vi "Open serial.vi"(8 "error in (no error)":errorcluster, 10 "port":string, 11 "Roda_Filtros in":refnum<class "Roda_Filtros.lvclass">) -> (0 "error out":errorcluster, 2 "status":bool, 3 "Roda_Filtros out":refnum<class "Roda_Filtros.lvclass">)   [LabVIEW 2018, in "Roda_Filtros.lvclass"]
uses:
  Roda_Filtros.lvclass
  Roda_Filtros.lvclass/Roda_Filtros.ctl
  <vilib>/Instr/_visa.llb/VISA Configure Serial Port (Instr).vi
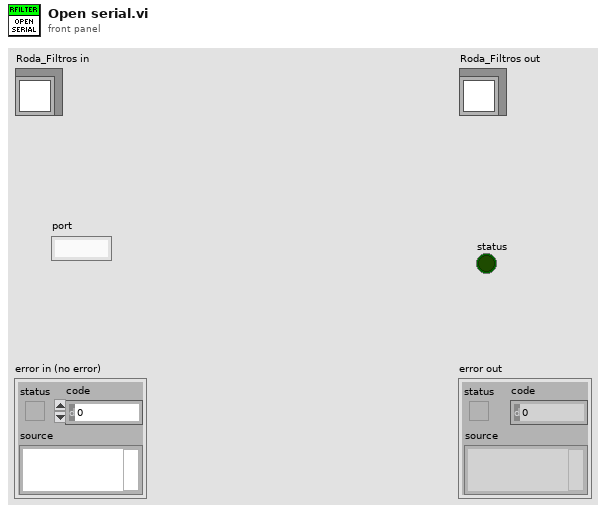
[diagram p1: front panel]
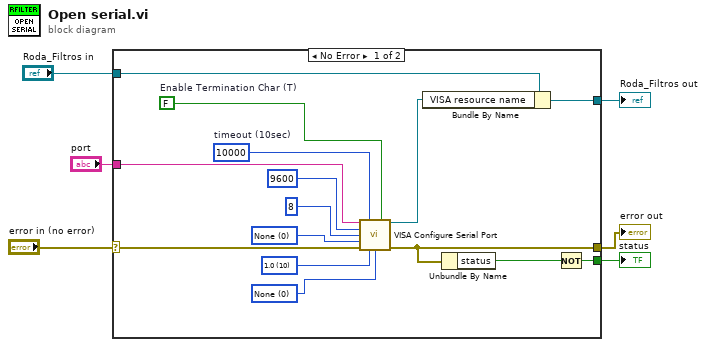
[diagram p0: block diagram]
diagram:
  n1 = case shown="No Error" "error in (no error)" {
    selector: "error in (no error)" -> [w14 w23]
    tunnel: [w9 w23] -> w5
    tunnel: [w12 w22] -> w3
    tunnel: "Roda_Filtros in" -> [w13 w22]
    tunnel: "port" -> [w10 _]
    tunnel: [w7 _] -> w1
    frame No Error {
      w20 = u16 0 items=["None", "Odd", "Even", "Mark", "Space"] ("parity")
      w17 = u16 10 items=["1.0"=10, "1.5"=15, "2.0"=20] ("stop bits")
      w16 = u16 0 items=["None"=0, "XON/XOFF"=1, "RTS/CTS"=2, "DTR/DSR"=4] ("flow control")
      w18 = FALSE  # Enable Termination Char (T)
      w19 = u32 10000  # timeout (10sec)
      n2 = call-poly "VISA Configure Serial Port"("VISA resource name"=w10, "timeout (10sec)"=w19, "Enable Termination\nChar (T)"=w18, "baud rate (9600)"=u32 9600 ("baud rate"), "data bits (8)"=u16 8 ("data bits"), "parity (0:none)"=w20, "error in (no error)"=w14, "stop bits (10: 1 bit)"=w17, "flow control (0:none)"=w16) -> ("VISA resource name out"=w11:refnum<visa-resource-name>, "error out"=w9:errorcluster)  [unwired: 5 in]
      n3 = Bundle By Name(cluster=w13, "VISA resource name"=w11) -> (w12:refnum<class "Roda_Filtros.lvclass">)
      n4 = Unbundle By Name(w9) -> ("status"=w8:bool)
      n5 = Not(x=w8) -> (.not. x?=w7:bool)
    }
    frame Error {
    }
  }
  "error out" <- w5
  "Roda_Filtros out" <- w3
  "status" <- w1
